vi "Vision Research Phantom Series PhInt PhWBAdjustUnint.vi"(0 "pBMIH":T3, 1 "pPixel in":u16[](array[numeric]), 3 "CFA":T2 {"CFA" items=["CFA_NONE", "CFA_VRI", "CFA_VRIV6", "CFA_BAYER", "CFA_BAYERFLIP"]}, 5 "Error In (no error)":errorcluster, 9 "WBGAIN":T1) -> (15 "pPixel out":u16[](array[numeric]), 19 "Error Out":errorcluster)   [LabVIEW 2013, in "VRI.lvlib"]
doc: "PhInt.dll\n\nPhWBAdjustUnint\nvoid PhWBAdjustUnint(PBITMAPINFOHEADER pBMIH, PBYTE pPixel, UINT CFA, PWBGAIN pWBg);\n\nParameters Description\npBMIH Source and destination header of the processed image.\npPixel Source and destination pixel array of the processed image.\nCFA Color filter array of the camera sensor used to acquire this image.\npWBg Gain corrections on red and blue components used to adjust the white balance.\nReturn void\nComments PhWBAdjustUnint applies gain corrections on the red and blue components of the \n pixels. It operates on an uninterpolated image read from the sensor or from an \n uninterpolated cine file. The result image is better if the White Balance correction\n is applied before interpolation. To apply White Balance corrections on interpolated\n images use the PhImProc function and the WBView field of the IMPROCOPTIONS\n structure."
uses:
  VRI.lvlib
  _Type Defs/BITMAPINFOHEADER.ctl
  _Type Defs/PhInt CFA.ctl
  _Type Defs/PhInt WBGAIN.ctl
  Phantom DLLs/PhInt.dll
panel:
  # "For instructions on the use of this VI, press Ctrl+H to display the help window and move the mouse over the icon, controls, and indicators"
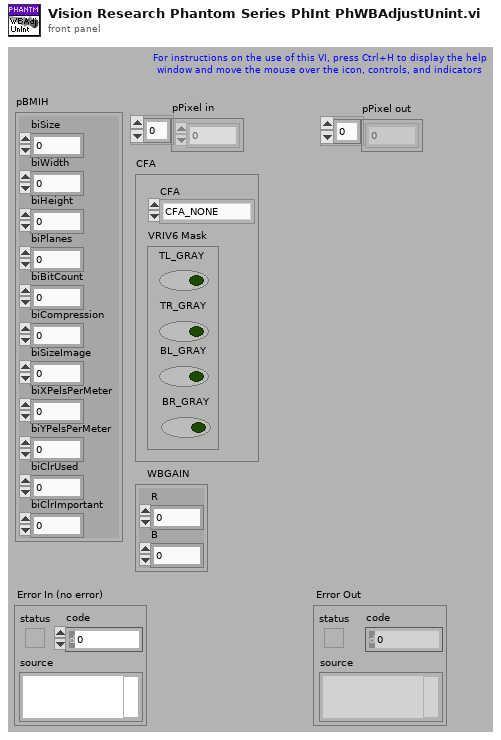
[diagram p1: front panel]
types:
  T1 = typedef "VRI.lvlib/PhInt WBGAIN.ctl" = cluster{"R":sgl, "B":sgl}
  T2 = typedef "VRI.lvlib/PhInt CFA.ctl" = cluster{"CFA":u32, "VRIV6 Mask":cluster{"TL_GRAY":bool, "TR_GRAY":bool, "BL_GRAY":bool, "BR_GRAY":bool}}
  T3 = typedef "VRI.lvlib/BITMAPINFOHEADER.ctl" = cluster{"biSize":u32, "biWidth":i32, "biHeight":i32, "biPlanes":u16, "biBitCount":u16, "biCompression":u32, "biSizeImage":u32, "biXPelsPerMeter":i32, "biYPelsPerMeter":i32, "biClrUsed":u32, "biClrImportant":u32}
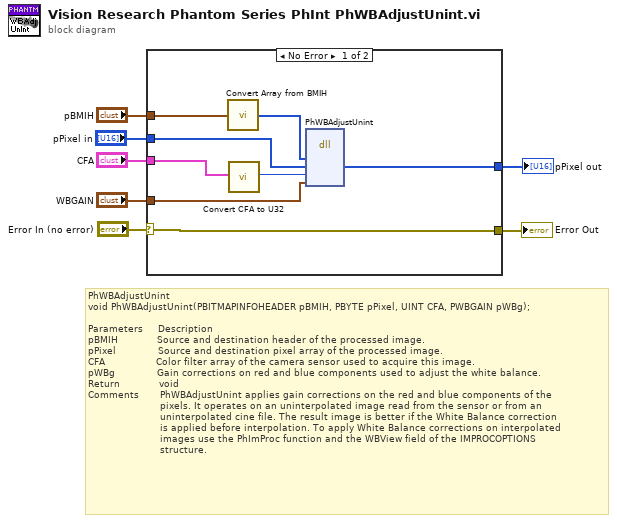
[diagram p0: block diagram]
diagram:
  # "PhWBAdjustUnint\nvoid PhWBAdjustUnint(PBITMAPINFOHEADER pBMIH, PBYTE pPixel, UINT CFA, PWBGAIN pWBg);\n\nParameters     Description\npBMIH             Source and destination header of the processed image.\npPixel              Source and destination pixel array of the processed image.\nCFA                 Color filter array of the camera sensor used to acquire this image.\npWBg              Gain corrections on red and blue components used to adjust the white balance.\nReturn             void\nComments       PhWBAdjustUnint applies gain corrections on the red and blue components of the \n                        pixels. It operates on an uninterpolated image read from the sensor or from an \n                        uninterpolated cine file. The result image is better if the White Balance correction\n                        is applied before interpolation. To apply White Balance corrections on interpolated\n                        images use the PhImProc function and the WBView field of the IMPROCOPTIONS\n                        structure."
  n1 = case shown="No Error" "Error In (no error)" {
    selector: "Error In (no error)" -> [w15 w17]
    tunnel: [w15 w17] -> w6
    tunnel: "pBMIH" -> [w14 _]
    tunnel: "CFA" -> [w13 _]
    tunnel: "pPixel in" -> [w12 w16]
    tunnel: [w11 w16] -> w2
    tunnel: "WBGAIN" -> [w10 _]
    frame No Error {
      n2 = call "Convert Array from BMIH.vi"("BITMAPINFOHEADER"=w14) -> ("Array"=w9:u8[])
      n3 = call "Convert CFA to U32.vi"("CFA in"=w13) -> ("CFA out"=w8:u32)  [unwired: 18 out]
      n4 = dll-call lib="C:/Projects/SDK/32-bit/Vision Research Phantom Series Labview Driver/Phantom DLLs/PhInt.dll" fn="PhWBAdjustUnint"("pBMIH"=w9, "pPixel"=w12, "CFA"=w8, "pWBg"=w10) -> ("pPixel"=w11:u16[])  [unwired: 6 in, 3 out]
    }
    frame Error {
    }
  }
  "Error Out" <- w6
  "pPixel out" <- w2
